vi "SelectorTallestTarget.vi"(0 "Array":T1(array[cluster])) -> (7 "VisionClusterOut":T2={"Position"={"X"=0.0, "Y"=0.0}, "Distance (ft)"=0.0, "NoTarget"=TRUE, "Right"=TRUE, "Center"=FALSE, "Left"=TRUE, "TargetCenter"=0.0})   [LabVIEW 2011]
panel:
  out "BetterDistanceV2 - Avg":dbl
  out "BetterDistanceMiddle":dbl
  out "BetterDistanceV1":dbl
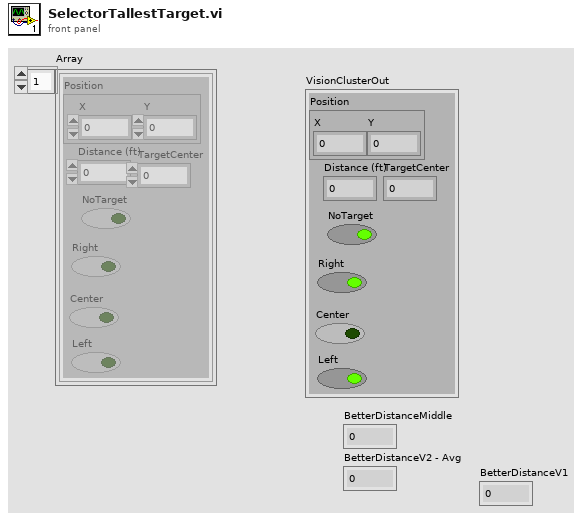
[diagram p1: front panel]
types:
  T1 = cluster{"Position":cluster{"X":dbl, "Y":dbl}, "Distance (ft)":dbl, "NoTarget":bool, "Right":bool, "Center":bool, "Left":bool, "TargetCenter":dbl}[]
  T2 = cluster{"Position":cluster{"X":dbl, "Y":dbl}, "Distance (ft)":dbl, "NoTarget":bool, "Right":bool, "Center":bool, "Left":bool, "TargetCenter":dbl}
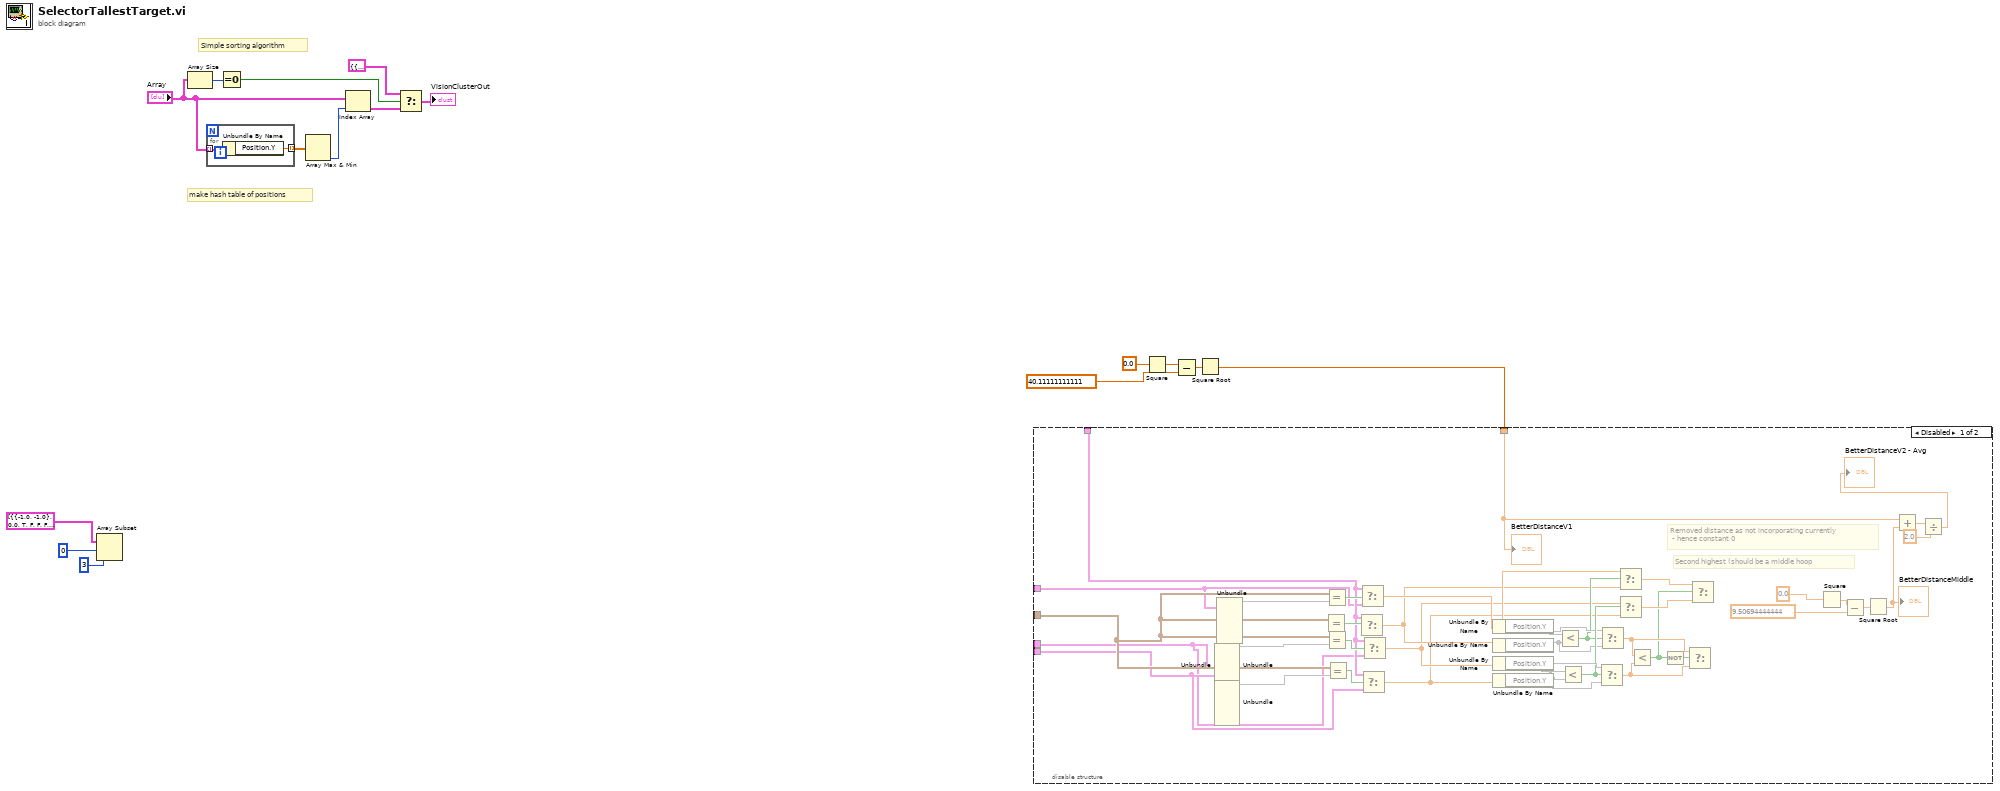
[diagram p0: block diagram]
diagram:
  # "Simple sorting algorithm"
  # "make hash table of positions"
  n1 = Array Subset(array=T1 [{"Position"={"X"=-1.0, "Y"=-1.0}, "Distance (ft)"=0.0, "NoTarget"=TRUE, "Right"=FALSE, "Center"=FALSE, "Left"=FALSE, "TargetCenter"=0.0}, {"Position"={"X"=0.0, "Y"=0.0}, "Distance (ft)"=16.0, "NoTarget"=FALSE, "Right"=FALSE, "Center"=FALSE, "Left"=TRUE, "TargetCenter"=0.0}, {"Position"={"X"=-0.234375, "Y"=0.5375}, "Distance (ft)"=14.583387907116473, "NoTarget"=FALSE, "Right"=TRUE, "Center"=TRUE, "Left"=FALSE, "TargetCenter"=-0.0234375}, {"Position"={"X"=-0.56875, "Y"=-0.1125}, "Distance (ft)"=16.71013197690429, "NoTarget"=FALSE, "Right"=TRUE, "Center"=FALSE, "Left"=FALSE, "TargetCenter"=-0.190625}] ("Array"), index=0, length=3) -> ()  [unwired: 1 out]
  n2 = Array Size(array="Array") -> (size(s)=w6:i32)
  n3 = for {
    tunnel: "Array" -> [w19] mode=indexing
    tunnel: [w18] -> w8 mode=indexing
    n4 = Unbundle By Name(w19) -> ("Position.Y"=w18:dbl)
  }
  n5 = Equal To 0?(x=w6) -> (x = 0?=w5:bool)
  n6 = Array Max & Min(array=w8) -> (min index (indices)=w7:i32)  [unwired: 3 out]
  n7 = Index Array(array="Array", index=w7) -> (element=w3:T2)
  n8 = Select(t=T2 {"Position"={"X"=0.0, "Y"=0.0}, "Distance (ft)"=0.0, "NoTarget"=TRUE, "Right"=TRUE, "Center"=FALSE, "Left"=TRUE, "TargetCenter"=0.0} ("VisionClusterOut"), s=w5, f=w3) -> (s? t:f=→"VisionClusterOut":T2)
  n9 = Square(x=0.0) -> (x^2=w14:dbl)
  n10 = Subtract(x=w14, y=40.11111111111) -> (x-y=w13:dbl)
  n11 = Square Root(x=w13) -> (sqrt(x)=w12:dbl)
  n12 = disable-structure shown="Disabled" {
    disable-tunnel: w12 -> [w38 _]
    disable-tunnel: _ -> [w27 _]
    disable-tunnel: [w24 _] -> w10
    disable-tunnel: _ -> [w23 _]
    disable-tunnel: _ -> [w22 _]
    disable-tunnel: _ -> [w20 _]
    frame Disabled {
      # "Removed distance as not incorporating currently\n - hence constant 0"
      # "Second highest (should be a middle hoop"
      n13 = Unbundle(w20) -> ("Position"=w21)  [unwired: 6 out]
      n14 = Unbundle(w22) -> ()  [unwired: 7 out]
      n15 = Unbundle(w23) -> ("Position"=w26)  [unwired: 6 out]
      n16 = Unbundle(w20) -> ("Position"=w25)  [unwired: 6 out]
      n17 = Equal?(x=w27) -> (x = y?=w55:bool)  [unwired: 1 in]
      n18 = Equal?(x=w27, y=w25) -> (x = y?=w56:bool)
      n19 = Equal?(x=w27, y=w21) -> (x = y?=w54:bool)
      n20 = Equal?(x=w27, y=w26) -> (x = y?=w53:bool)
      n21 = Select(t=w24, s=w55) -> (s? t:f=w31:dbl)  [unwired: 1 in]
      n22 = Select(t=w24, s=w56, f=w20) -> (s? t:f=w32:dbl)
      n23 = Select(t=w24, s=w53, f=w23) -> (s? t:f=w29:dbl)
      n24 = Select(t=w24, s=w54, f=w22) -> (s? t:f=w30:dbl)
      n25 = Unbundle By Name(w32) -> ("Position.Y"=w44)
      n26 = Unbundle By Name(w31) -> ("Position.Y"=w43)
      n27 = Unbundle By Name(w30) -> ("Position.Y"=w49)
      n28 = Unbundle By Name(w29) -> ("Position.Y"=w48)
      n29 = Less?(x=w44, y=w43) -> (x < y?=w42:bool)
      n30 = Less?(x=w49, y=w48) -> (x < y?=w45:bool)
      n31 = Select(t=w49, s=w45, f=w48) -> (s? t:f=w51:dbl)
      n32 = Select(t=w44, s=w42, f=w43) -> (s? t:f=w50:dbl)
      n33 = Select(t=w32, s=w42, f=w31) -> (s? t:f=w46:dbl)
      n34 = Select(t=w30, s=w45, f=w29) -> (s? t:f=w47:dbl)
      n35 = Less?(x=w50, y=w51) -> (x < y?=w33:bool)
      n36 = Not(x=w33) -> (.not. x?=w52:bool)
      n37 = Select(t=w50, s=w52, f=w51) -> ()  [unwired: 1 out]
      n38 = Select(t=w46, s=w33, f=w47) -> ()  [unwired: 1 out]
      n39 = Square(x=0.0) -> (x^2=w40:dbl)
      n40 = Subtract(x=w40, y=9.50694444444) -> (x-y=w41:dbl)
      n41 = Square Root(x=w41) -> (sqrt(x)=w37:dbl)
      "BetterDistanceMiddle" <- w37
      n42 = Add(x=w38, y=w37) -> (x+y=w36:dbl)
      n43 = Divide(x=w36, y=2.0) -> (x/y=→"BetterDistanceV2 - Avg":dbl)
      "BetterDistanceV1" <- w38
    }
    frame Enabled {
    }
  }
